vi "Set_Display_Path.vi"(8 "error in (no error)":errorcluster, 10 "displayPath":path, 11 "AB_Dest_App in":refnum<class "AB_Dest_LegacyApp.lvclass">) -> (0 "error out":errorcluster, 3 "AB_Dest_App out":refnum<class "AB_Dest_LegacyApp.lvclass">)   [LabVIEW 2020, in "AB_Dest_LegacyApp.lvclass"]
uses:
  <vilib>/AppBuilder/AB_Classes/Destination/Dest_LegacyApplication/AB_Dest_LegacyApp.lvclass
  e:/builds/penguin/labview/branches/2020/dev/dist/vi.lib/AppBuilder/AB_Classes/Destination/AB_Destination.lvclass
  <vilib>/AppBuilder/AB_Classes/Destination/AB_Destination.lvclass
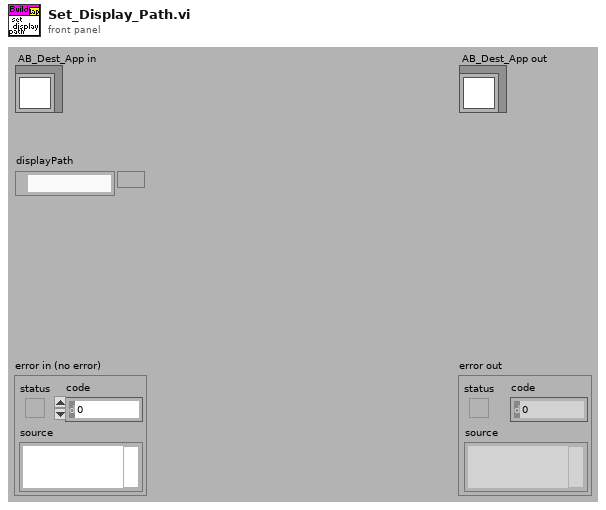
[diagram p1: front panel]
types:
  T1 = typedef "AB_Destination.ctl" = cluster{"destName":string, "path":path, "libraryName":string, "preserveHierarchy":bool, "eng_inBuild":bool, "eng_libraryReference":refnum<vi>, "eng_restictAddToNewLibrary":bool}
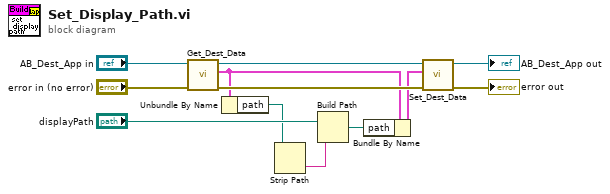
[diagram p0: block diagram]
diagram:
  n1 = call <vilib>:"Get_Dest_Data.vi"("error in (no error)"="error in (no error)", "Class in"="AB_Dest_App in") -> ("error out"=w6:errorcluster, "destName"=w3:T1, "Class out"=w9:refnum<class "AB_Dest_LegacyApp.lvclass">)  [unwired: 7 out]
  n2 = Unbundle By Name(w3) -> ("path"=w4:path)
  n3 = Strip Path(path=w4) -> (name=w12:string)  [unwired: 1 out]
  n4 = Build Path(base path="displayPath", name or relative path=w12) -> (appended path=w1:path)
  n5 = Bundle By Name(cluster=w3, "path"=w1) -> (w2:T1)
  n6 = call <vilib>:"Set_Dest_Data.vi"("error in (no error)"=w6, "destName"=w2, "Class in"=w9) -> ("error out"=→"error out":errorcluster, "Class out"=→"AB_Dest_App out":refnum<class "AB_Dest_LegacyApp.lvclass">)  [unwired: 7 out]
